vi "GetData.vi"(8 "error in (no error)":errorcluster, 11 "Electrophysiology in":refnum<class "Electrophysiology.lvclass">) -> (0 "error out":errorcluster, 1 "Samples":dbl, 2 "data":waveform(dbl)[](array[waveform]), 3 "Electrophysiology out":refnum<class "Electrophysiology.lvclass">)   [LabVIEW 2010, in "Electrophysiology.lvclass"]
uses:
  Electrophysiology.lvclass
  Electrophysiology.lvclass/Electrophysiology.ctl
  <vilib>/DAQmx/read.llb/DAQmx Read (Analog 1D Wfm NChan NSamp).vi
  <vilib>/daqmx/miscellaneous.llb/DAQmx Fill In Error Info.vi
  Program Files/National Instruments/LabVIEW 2010/resource/objmgr/daqmx.rc
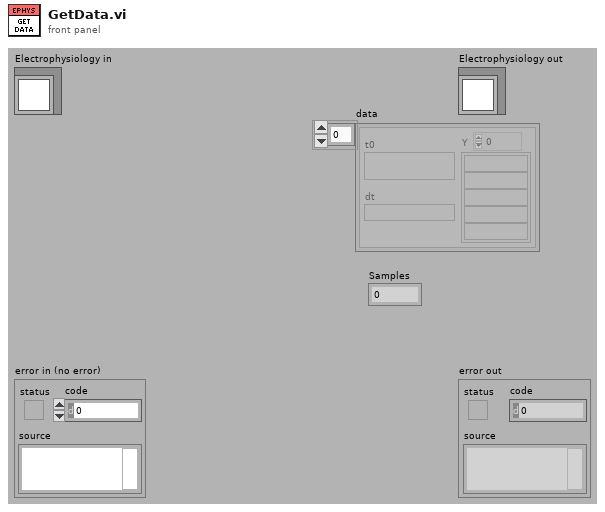
[diagram p1: front panel]
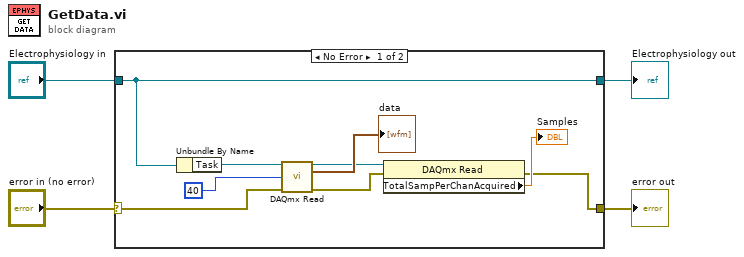
[diagram p0: block diagram]
diagram:
  n1 = case shown="No Error" "error in (no error)" {
    selector: "error in (no error)" -> [w10 w15]
    tunnel: [w5 w15] -> w3
    tunnel: [w13 w14] -> w1
    tunnel: "Electrophysiology in" -> [w13 w14]
    frame No Error {
      n2 = Unbundle By Name(w13) -> ("Task"=w11:refnum<k21>)
      n3 = call-poly <vilib>:"DAQmx Read.vi"("task/channels in"=w11, "number of samples per channel"=40, "error in"=w10) -> ("task out"=w7:refnum<k21>, "data"=→"data":waveform(dbl)[], "error out"=w6:errorcluster)  [unwired: 10 in]
      n4 = property class="DAQmx Read"(reference=w7, error in=w6) -> (error out=w5:errorcluster, "TotalSampPerChanAcquired"=→"Samples":dbl)  [unwired: 1 out]
    }
    frame Error {
    }
  }
  "error out" <- w3
  "Electrophysiology out" <- w1
